vi "MultiChannnel_With_Origin_init_Matrix.vi"() -> ()   [LabVIEW 2024]
uses:
  <vilib>/DAQmx/read.llb/DAQmx Read (Analog 1D Wfm NChan NSamp).vi
  <vilib>/Analysis/baseanly.llb/Real A x B.vi
  <vilib>/Analysis/baseanly.llb/Mean (DBL).vi
  <vilib>/DAQmx/create/channels.llb/DAQmx Create Channel (AI-Voltage-Basic).vi
  <vilib>/DAQmx/configure/timing.llb/DAQmx Timing (Sample Clock).vi
  <vilib>/DAQmx/miscellaneous.llb/DAQmx Fill In Error Info.vi
  <vilib>/Waveform/WDTOps.llb/WDT Index Channel DBL.vi
  <vilib>/Analysis/Matrix/Numeric/Conversions/Matrix To Array - RM.vi
  <vilib>/Analysis/NI_AALBase.lvlib
  <vilib>/Analysis/Matrix/NI_Matrix.lvlib
panel:
  out "Force Graph":dbl[][](graph)
  out "Force Array (F)   -> Time":dbl[][](array[numeric]) format="%#.3f"
  in  "Convert Matrix":dbl[][](array[numeric])=[[0.01787384, 0.5614992, -0.6825333], [-0.80829626, 0.31005788, 0.3553213], [0.6880116, 0.4358145, 0.7359737]]
  in  "StopAll":bool
  out "How many time get offset":i32
  out "Ch3 Origin":dbl
  out "Ch2 Origin":dbl
  out "Ch1 Origin":dbl
  out "RawCantilever (V) (Offset removed     -> Time)":dbl[][](array[numeric]) format="%#.3f"
  out "C 3":dbl[](array[numeric]) format="%#.5g"
  out "C 2":dbl[](array[numeric]) format="%#.5g"
  out "C1":dbl[](array[numeric]) format="%#.5g"
  in  "Get Orogin":bool
  out "Raw AD":waveform(dbl)[](graph)
  in  "samples per channel":i32=500
  in  "sample mode":i32(ring)=10123 items=["Continuous Samples"=10123, "Finite Samples"=10178, "Hardware Timed Single Point"=12522]
  in  "rate":dbl=1000.0 format="%0.2f"
  in  "physical channels":tag="Dev2/ai0:2"
  # "Phy Channel -> Set to 0-2\nRate 1000Hz\nSampleMode  -> Contenious Sampling\nSample per Channel -> 100"
  # "Raw A/D (V)"
  # "C1"
  # "Shear X"
  # "C2"
  # "Shear Y"
  # "Offset (V)"
  # "C3"
  # "Force Z"
  # "No.509 \n[[ 0.01787384, 0.5614992 , -0.6825333 ],\n[-0.80829626, 0.31005788, 0.3553213 ],\n[ 0.6880116 , 0.4358145 , 0.7359737 ]"
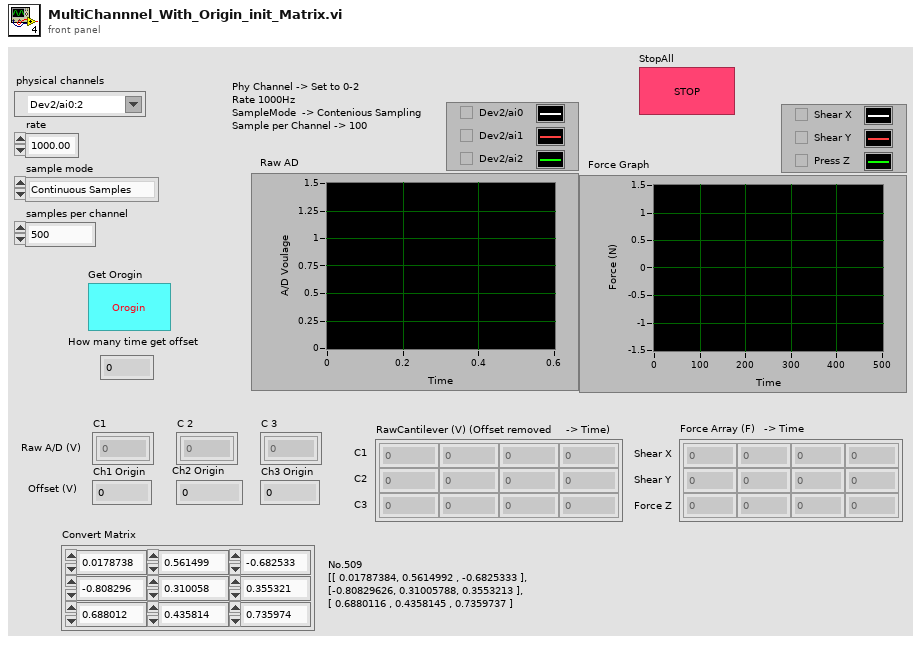
[diagram p1: front panel]
types:
  T1 = typedef "NI_Matrix.lvlib/RealMatrix.ctl" = dbl[][]
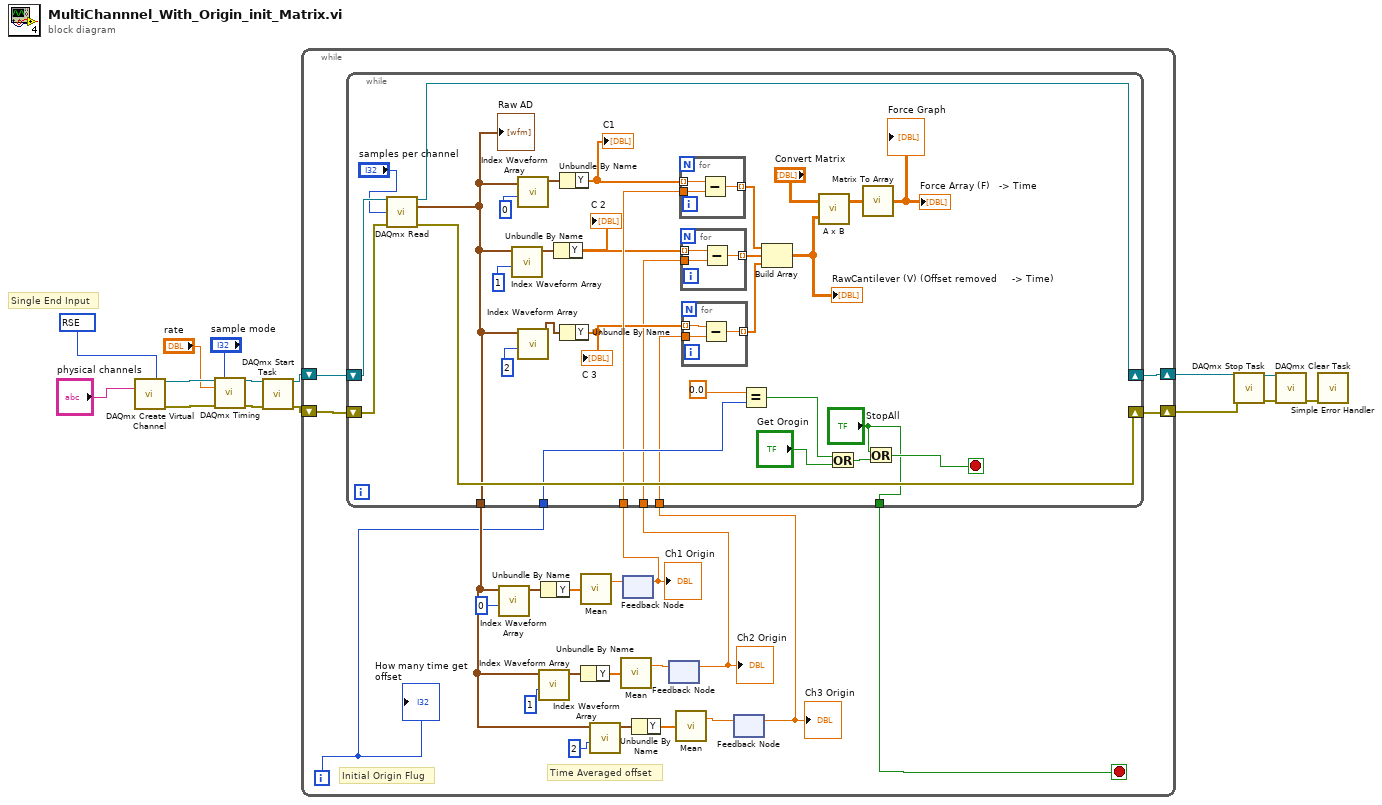
[diagram p0: block diagram]
diagram:
  w1 = 10083 items=["Default"=-1, "RSE"=10083, "NRSE"=10078, "Differential"=10106, "Pseudodifferential"=12529] ("input terminal configuration")
  # "Single End Input"
  n1 = call-poly <vilib>:"DAQmx Create Virtual Channel.vi"("input terminal configuration"=w1, "physical channels"="physical channels") -> ("task out"=w7:refnum<k21>, "error out"=w6:errorcluster)  [unwired: 12 in]
  n2 = call-poly <vilib>:"DAQmx Timing.vi"("task/channels in"=w7, "sample mode"="sample mode", "rate"="rate", "error in"=w6) -> ("task out"=w5:refnum<k21>, "error out"=w4:errorcluster)  [unwired: 10 in]
  n3 = call <vilib>:"DAQmx Start Task.vi"("task/channels in"=w5, "error in"=w4) -> ("task out"=w14:refnum<k21>, "error out"=w13:errorcluster)  [unwired: 12 in]
  n4 = while {
    shift-right: [w34] -> w11
    shift-left: w14 -> [w37]
    shift-right: [w35] -> w12
    shift-left: w13 -> [w36]
    i -> [w25]
    stop <- w26 stop-if-true
    # "Time Averaged offset"
    # "Initial Origin Flug"
    n5 = feedback #1() -> (w21:dbl)  [unwired: 1 in]
    "Ch1 Origin" <- w21
    n6 = feedback #2() -> (w16:dbl)  [unwired: 1 in]
    "Ch2 Origin" <- w16
    n7 = feedback #3() -> (w17:dbl)  [unwired: 1 in]
    "Ch3 Origin" <- w17
    n8 = while {
      shift-right: [w66] -> w34
      shift-left: w37 -> [w69]
      shift-right: [w67] -> w35
      shift-left: w36 -> [w68]
      tunnel: [w38] -> w30
      tunnel: ["StopAll"] -> w26
      tunnel: w25 -> [w55]
      tunnel: w21 -> [w47]
      tunnel: w16 -> [w43]
      tunnel: w17 -> [w42]
      stop <- w58 stop-if-true
      n9 = call-poly <vilib>:"DAQmx Read.vi"("task/channels in"=w69, "number of samples per channel"="samples per channel", "error in"=w68) -> ("task out"=w66:refnum<k21>, "data"=w38:waveform(dbl)[], "error out"=w67:errorcluster)  [unwired: 10 in]
      "Raw AD" <- w38
      n10 = call-poly <vilib>:"Index Waveform Array.vi"("index"=1, "waveform array"=w38) -> ("waveform"=w61:waveform(dbl))  [unwired: 8 in, 1 out]
      n11 = call-poly <vilib>:"Index Waveform Array.vi"("index"=0, "waveform array"=w38) -> ("waveform"=w63:waveform(dbl))  [unwired: 8 in, 1 out]
      n12 = call-poly <vilib>:"Index Waveform Array.vi"("index"=2, "waveform array"=w38) -> ("waveform"=w59:waveform(dbl))  [unwired: 8 in, 1 out]
      n13 = Unbundle By Name(w61) -> ("Y"=w45:dbl[])
      "C 2" <- w45
      n14 = Unbundle By Name(w63) -> ("Y"=w48:dbl[])
      "C1" <- w48
      n15 = Unbundle By Name(w59) -> ("Y"=w44:dbl[])
      "C 3" <- w44
      n16 = for {
        tunnel: w48 -> [w78] mode=indexing
        tunnel: w47 -> [w77]
        tunnel: [w76] -> w46 mode=indexing
        n17 = Subtract(x=w78, y=w77) -> (x-y=w76:dbl)
      }
      n18 = for {
        tunnel: [w75] -> w41 mode=indexing
        tunnel: w45 -> [w74] mode=indexing
        tunnel: w43 -> [w73]
        n19 = Subtract(x=w74, y=w73) -> (x-y=w75:dbl)
      }
      n20 = for {
        tunnel: [w72] -> w40 mode=indexing
        tunnel: w44 -> [w71] mode=indexing
        tunnel: w42 -> [w70]
        n21 = Subtract(x=w71, y=w70) -> (x-y=w72:dbl)
      }
      n22 = Equal?(x=0.0, y=w55) -> (x = y?=w54:bool)
      n23 = Build Array(w46, w41, w40) -> (w49:dbl[][])
      "RawCantilever (V) (Offset removed     -> Time)" <- w49
      n24 = call-poly <vilib>:"A x B.vi"("B"=w49, "A"="Convert Matrix") -> ("A x B"=w51:T1)  [unwired: 1 out]
      n25 = Or(x=w54, y="Get Orogin") -> (x .or. y?=w52:bool)
      n26 = call-poly <vilib>:"Matrix To Array.vi"("Real Matrix"=w51) -> ("Real 2D Array"=→"Force Array (F)   -> Time" →"Force Graph":dbl[][])
      n27 = Or(x="StopAll", y=w52) -> (x .or. y?=w58:bool)
    }
    n28 = call-poly <vilib>:"Index Waveform Array.vi"("index"=0, "waveform array"=w30) -> ("waveform"=w33:waveform(dbl))  [unwired: 8 in, 1 out]
    n29 = call-poly <vilib>:"Index Waveform Array.vi"("index"=1, "waveform array"=w30) -> ("waveform"=w32:waveform(dbl))  [unwired: 8 in, 1 out]
    n30 = Unbundle By Name(w33) -> ("Y"=w24:dbl[])
    n31 = call-poly <vilib>:"Mean.vi"("X"=w24) -> ("mean"=w22:dbl)  [unwired: 1 out]
    n32 = Unbundle By Name(w32) -> ("Y"=w23:dbl[])
    n33 = call-poly <vilib>:"Index Waveform Array.vi"("index"=2, "waveform array"=w30) -> ("waveform"=w31:waveform(dbl))  [unwired: 8 in, 1 out]
    n34 = call-poly <vilib>:"Mean.vi"("X"=w23) -> ("mean"=w20:dbl)  [unwired: 1 out]
    n35 = feedback-in #1(w22) -> ()
    n36 = Unbundle By Name(w31) -> ("Y"=w19:dbl[])
    n37 = feedback-in #2(w20) -> ()
    n38 = call-poly <vilib>:"Mean.vi"("X"=w19) -> ("mean"=w18:dbl)  [unwired: 1 out]
    n39 = feedback-in #3(w18) -> ()
    "How many time get offset" <- w25
  }
  n40 = call <vilib>:"DAQmx Stop Task.vi"("task/channels in"=w11, "error in"=w12) -> ("task out"=w9:refnum<k21>, "error out"=w10:errorcluster)  [unwired: 12 in]
  n41 = call <vilib>:"DAQmx Clear Task.vi"("task in"=w9, "error in"=w10) -> ("error out"=w8:errorcluster)  [unwired: 13 in]
  n42 = call <vilib>:"Simple Error Handler.vi"("error in (no error)"=w8) -> ()  [unwired: 4 in, 5 out]
